vi "make.vi"(8 "error in (no error)":errorcluster, 11 "MultiUsrp in":refnum<class "MultiUsrp.lvclass">) -> (0 "error out":errorcluster, 3 "MultiUsrp out":refnum<class "MultiUsrp.lvclass">)   [LabVIEW 2023, in "uhd.lvlib" / "MultiUsrp.lvclass"]
uses:
  <userlib>/uhd/MultiUsrp/MultiUsrp.lvclass
  <userlib>/uhd/MultiUsrp/MultiUsrp.lvclass/MultiUsrp.ctl
  <userlib>/uhd/uhd.lvlib
panel:
  in  "args":string
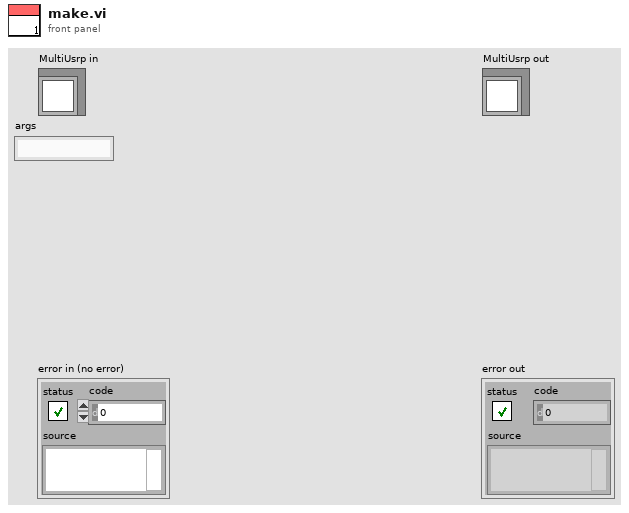
[diagram p1: front panel]
types:
  T1 = typedef "usrp session.ctl" = cluster{"h":u64, "Enum":enum16{"usrp handle"}}
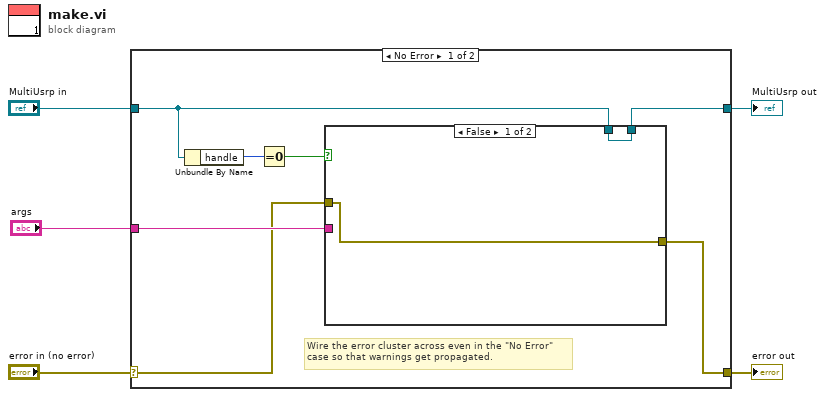
[diagram p0: block diagram]
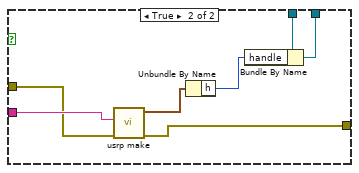
[diagram p2: hidden frame]
diagram:
  n1 = case shown="No Error" "error in (no error)" {
    selector: "error in (no error)" -> [w7 w23]
    tunnel: [w6 w23] -> w4
    tunnel: [w11 w22] -> w2
    tunnel: "MultiUsrp in" -> [w10 w22]
    tunnel: "args" -> [w12 _]
    frame No Error {
      # "Wire the error cluster across even in the \"No Error\"\ncase so that warnings get propagated."
      n2 = Unbundle By Name(w10) -> ("handle"=w9:u64)
      n3 = Equal To 0?(x=w9) -> (x = 0?=w8:bool)
      n4 = case shown="False" w8 {
        tunnel: w12 -> [_ w21]
        tunnel: [w14 w20] -> w11
        tunnel: w10 -> [w14 w17]
        tunnel: w7 -> [w13 w16]
        tunnel: [w13 w15] -> w6
        frame False {
        }
        frame True {
          n5 = call <userlib>:"usrp make.vi"("error in (no error)"=w16, "args"=w21) -> ("error out"=w15:errorcluster, "h 2"=w19:T1)  [unwired: 7 in, 1 out]
          n6 = Unbundle By Name(w19) -> ("h"=w18:u64)
          n7 = Bundle By Name(cluster=w17, "handle"=w18) -> (w20:refnum<class "MultiUsrp.lvclass">)
        }
      }
    }
    frame Error {
    }
  }
  "error out" <- w4
  "MultiUsrp out" <- w2
